vi "simulation.vi"(6 "stop":bool) -> ()   [LabVIEW 2010]
uses:
  red_tweezers_globals_INTERNAL.vi
  red_tweezers_globals.vi
  red_tweezers_globals_INTERNAL_VOLATILE.vi
  simulation_globals.vi
  <vilib>/Analysis/NI_AALBase.lvlib
panel:
  out "Image Out":T1(plugin-control)
  in  "timestep/s":dbl=0.009999999999999997 format="%.2p"
  in  "sedimentation velocity (m/s)":dbl=5e-07
  in  "trap autocorrelation time (s)":dbl=0.01
  in  "capture radius (m)":dbl=3e-06
  in  "diffusion (m/sqrt(s))":dbl=4e-07 format="%.2p"
  in  "Number of Particles":i32=10
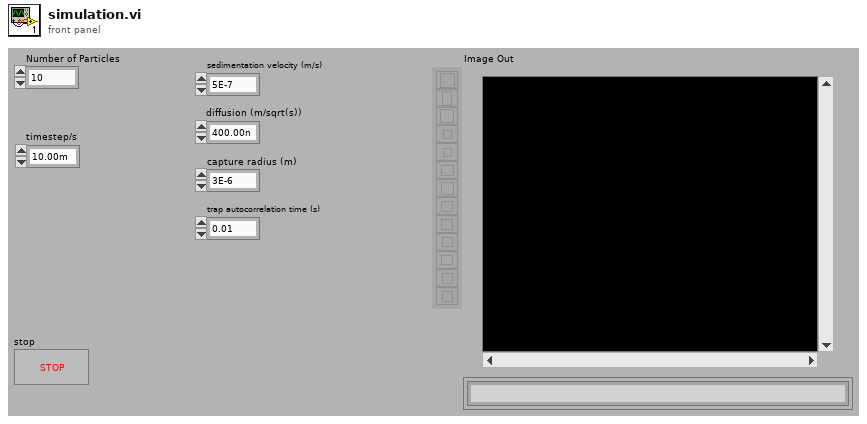
[diagram p1: front panel]
types:
  T1 = typedef "IMAQ Image.ctl" = refnum<image>
  T2 = enum32{"Bad", "Idle", "Run top level", "Running"}
  T3 = typedef "spot.ctl" = cluster{"Position":cluster{"x":dbl, "y":dbl, "z":dbl}, "Intensity":dbl, "Vortex Charge":i8, "Phase":dbl, "NA Position":cluster{"x":dbl, "y":dbl, "r":dbl}, "Line Trapping":T4, "Amplitude Correction":dbl}
  T4 = typedef "line_trapping.ctl" = cluster{"Vector":cluster{"x":dbl, "y":dbl, "z":dbl}, "Phase Gradient":dbl}
  T5 = cluster{"number: 0 to 1":dbl, "number: 0 to 1":dbl, "number: 0 to 1":dbl}
  T6 = cluster{"Gaussian noise pattern[0]":dbl, "Gaussian noise pattern[1]":dbl, "Gaussian noise pattern[2]":dbl}
  T7 = cluster{"capture radius":dbl, "capture radius":dbl, dbl}
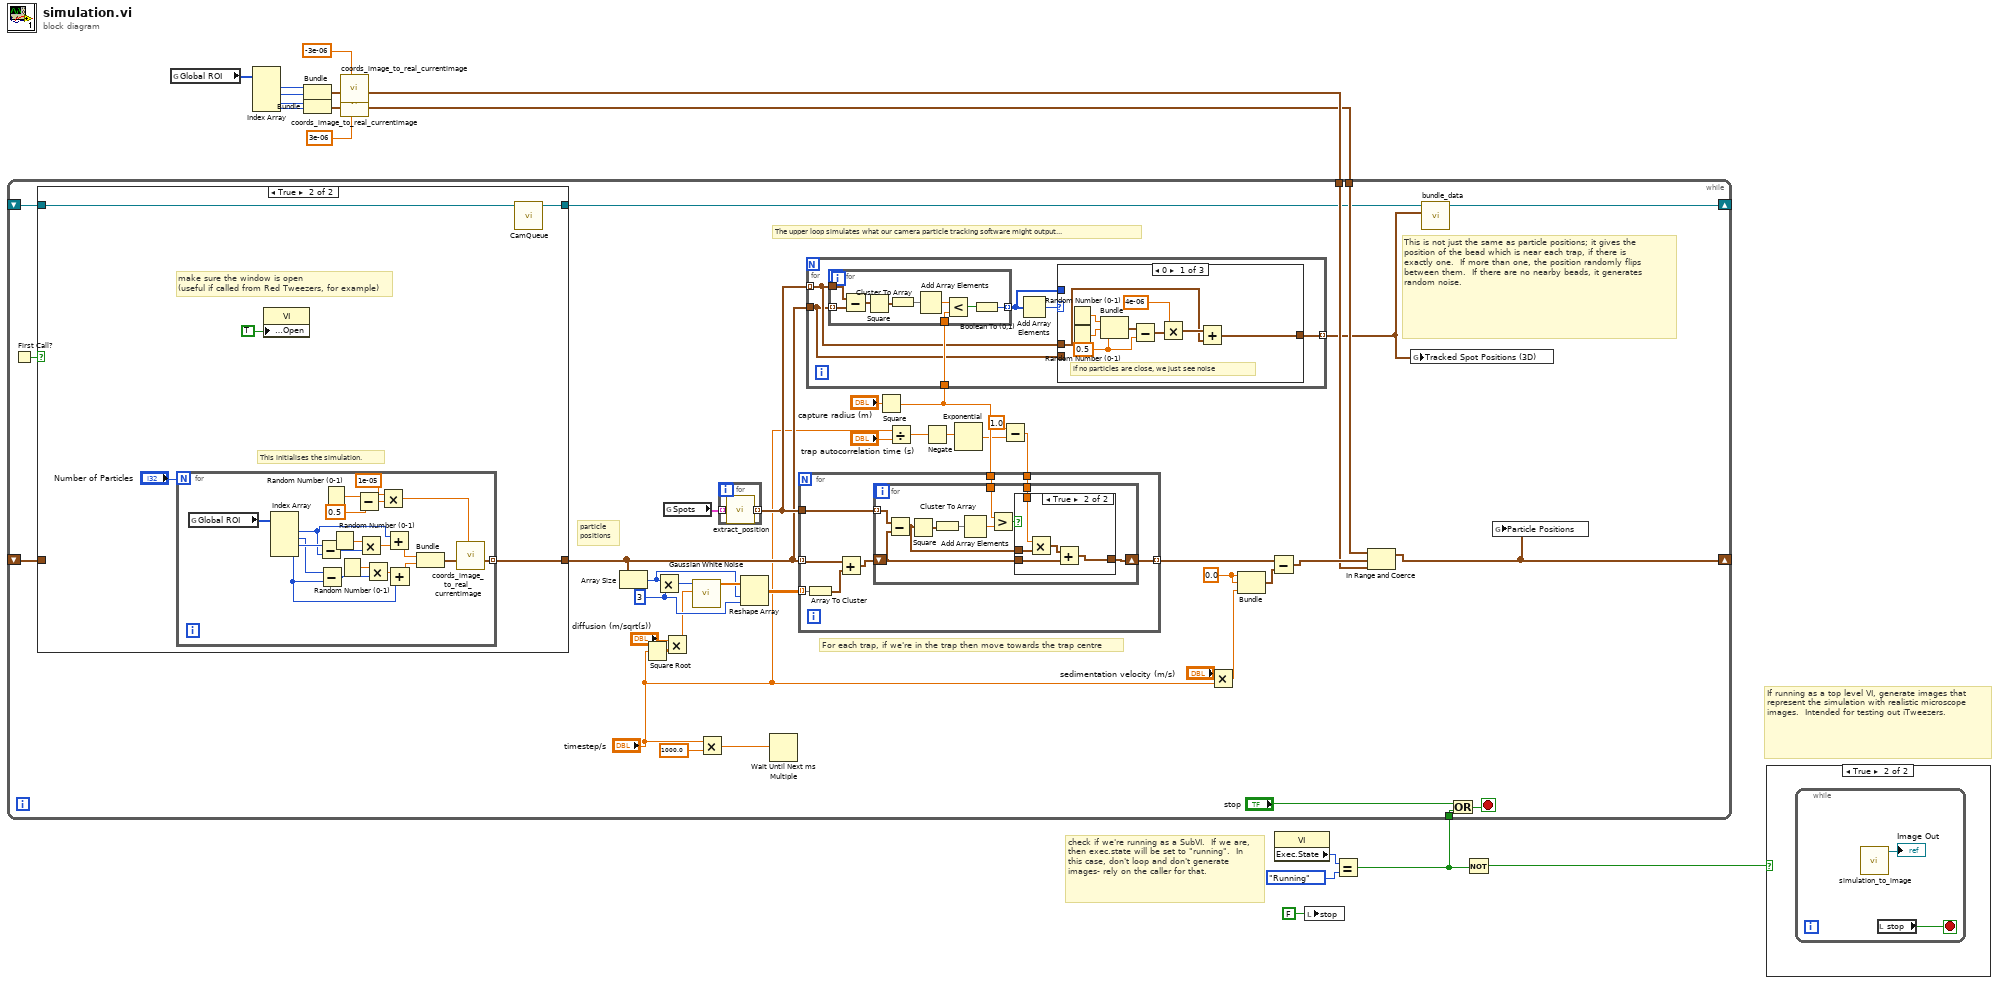
[diagram p0: block diagram]
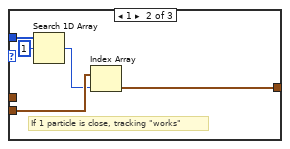
[diagram p4: hidden frame]
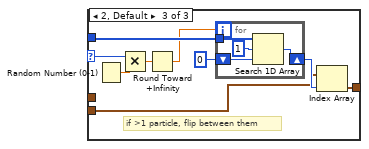
[diagram p5: hidden frame]
diagram:
  # "If running as a top level VI, generate images that represent the simulation with realistic microscope images.  Intended for testing out iTweezers."
  # "check if we're running as a SubVI.  If we are, then exec.state will be set to \"running\".  In this case, don't loop and don't generate images- rely on the caller for that."
  n1 = global read "red_tweezers_globals_INTERNAL.vi" "Global ROI"() -> (w16:i32[])
  n2 = Index Array(array=w16) -> (element #1=w15:i32, element #2=w14:i32, element #3=w9:i32, element #4=w8:i32)  [unwired: 4 in]
  n3 = Bundle("Numeric"=w15, "Numeric"=w14) -> (w13:cluster{"Numeric":i32, "Numeric":i32})  [unwired: 1 in]
  n4 = Bundle("Numeric"=w9, "Numeric"=w8) -> (w10:cluster{"Numeric":i32, "Numeric":i32})  [unwired: 1 in]
  n5 = call "coords_image_to_real_currentimage.vi"("Position (pixels on image)"=w13, "z (real coords)"=-3e-06) -> ("Position (real coords)"=w7:cluster{dbl, dbl, "Z":dbl})  [unwired: 8 in]
  n6 = call "coords_image_to_real_currentimage.vi"("Position (pixels on image)"=w10, "z (real coords)"=3e-06) -> ("Position (real coords)"=w6:cluster{dbl, dbl, "Z":dbl})  [unwired: 8 in]
  n7 = property class="VI"() -> ("Exec.State"=w5:T2)  [unwired: 2 in, 2 out]
  n8 = local write "stop"(FALSE ("stop")) -> ()
  n9 = Equal?(x=w5, y=T2."Running" ("Execution:State")) -> (x = y?=w2:bool)
  n10 = while {
    shift-right: [w44] -> _
    shift-left: _ -> [w29]
    tunnel: w7 -> [w43]
    tunnel: w6 -> [w42]
    shift-right: [w33] -> _
    shift-left: _ -> [w28]
    tunnel: w2 -> [w24]
    stop <- w26 stop-if-true
    w48 = 0.0 ("capture radius")
    w52 = 3 ("y")
    # "particle\npositions"
    # "This is not just the same as particle positions; it gives the position of the bead which is near each trap, if there is exactly one.  If more than one, the position randomly flips between them.  If there are no nearby beads, it generates random noise."
    # "The upper loop simulates what our camera particle tracking software might output..."
    # "For each trap, if we're in the trap then move towards the trap centre"
    n11 = First Call?() -> (First Call?: T/F=w27:bool)
    n12 = case shown="True" w27 {
      tunnel: [w57 w61] -> w30
      tunnel: [w56 w59] -> _
      tunnel: w29 -> [w57 _]
      tunnel: w28 -> [w56 _]
      frame False {
      }
      frame True {
        # "make sure the window is open\n(useful if called from Red Tweezers, for example)"
        # "This initialises the simulation."
        n13 = for {
          N: "Number of Particles" -> [_]
          tunnel: [w62] -> w61 mode=indexing
          n14 = global read "red_tweezers_globals_INTERNAL.vi" "Global ROI"() -> (w81:i32[])
          n15 = Index Array(array=w81) -> (element #1=w75:i32, element #2=w79:i32, element #3=w80:i32, element #4=w71:i32)  [unwired: 4 in]
          n16 = Subtract(x=w80, y=w75) -> (x-y=w78:i32)
          n17 = Subtract(x=w79, y=w71) -> (x-y=w73:i32)
          n18 = Random Number (0-1)() -> (number: 0 to 1=w67:dbl)
          n19 = Random Number (0-1)() -> (number: 0 to 1=w76:dbl)
          n20 = Random Number (0-1)() -> (number: 0 to 1=w74:dbl)
          n21 = Subtract(x=w67, y=0.5) -> (x-y=w65:dbl)
          n22 = Multiply(x=w76, y=w78) -> (x*y=w77:dbl)
          n23 = Multiply(x=w74, y=w73) -> (x*y=w72:dbl)
          n24 = Multiply(x=1e-05, y=w65) -> (x*y=w63:dbl)
          n25 = Add(x=w75, y=w77) -> (x+y=w69:dbl)
          n26 = Add(x=w72, y=w71) -> (x+y=w70:dbl)
          n27 = Bundle(w69, w70) -> (w68:cluster{dbl, dbl})  [unwired: 1 in]
          n28 = call "coords_image_to_real_currentimage.vi"("Position (pixels on image)"=w68, "z (real coords)"=w63) -> ("Position (real coords)"=w62:cluster{dbl, dbl, "Z":dbl})  [unwired: 8 in]
        }
        n29 = property class="VI"("Front Panel.Open"=TRUE ("Front Panel Window:Open")) -> ()  [unwired: 2 in, 2 out]
        n30 = call "CamQueue.vi"() -> ("queue out"=w59:refnum<queue>)  [unwired: 3 in]
      }
    }
    n31 = Array Size(array=w30) -> (size(s)=w53:i32)
    n32 = Square Root(x="timestep/s") -> (sqrt(x)=w39:dbl)
    n33 = Multiply(x=w53, y=w52) -> (x*y=w55:i32)
    n34 = Multiply(x="diffusion (m/sqrt(s))", y=w39) -> (x*y=w41:dbl)
    n35 = global read "red_tweezers_globals.vi" "Spots"() -> (w50:T3[])
    n36 = call <vilib>:"Gaussian White Noise.vi"("standard deviation"=w41, "samples"=w55) -> ("Gaussian noise pattern"=w54:dbl[])  [unwired: 8 in, 1 out]
    n37 = Multiply(x="timestep/s", y=1000.0) -> (x*y=w37:dbl)
    n38 = for {
      tunnel: w50 -> [w125] mode=indexing
      tunnel: [w124] -> w35 mode=indexing
      n39 = call "extract_position.vi"("Spot"=w125) -> ("Position"=w124:cluster{"x":dbl, "y":dbl, "z":dbl})
    }
    n40 = Reshape Array(w54, w53, w52) -> (w51:dbl[][])
    n41 = Wait Until Next ms Multiple(millisecond multiple=w37) -> ()  [unwired: 1 out]
    n42 = Square(x="capture radius (m)") -> (x^2=w31:dbl)
    n43 = for {
      tunnel: w35 -> [w85] mode=indexing
      tunnel: w30 -> [w84]
      tunnel: w31 -> [w87]
      tunnel: [w82] -> w32 mode=indexing
      n44 = for {
        tunnel: w85 -> [w123]
        tunnel: w84 -> [w118] mode=indexing
        tunnel: w87 -> [w117]
        tunnel: [w115] -> w83 mode=indexing
        n45 = Subtract(x=w123, y=w118) -> (x-y=w119:cluster{dbl, dbl, dbl})
        n46 = Square(x=w119) -> (x^2=w122:cluster{dbl, dbl, dbl})
        n47 = Cluster To Array(cluster=w122) -> (array=w121:dbl[])
        n48 = Add Array Elements(numeric array=w121) -> (sum=w120:dbl)
        n49 = Less?(x=w120, y=w117) -> (x < y?=w116:bool)
        n50 = Boolean To (0,1)(Boolean=w116) -> (0, 1=w115:i16)
      }
      n51 = Add Array Elements(numeric array=w83) -> (sum=w86:i16)
      n52 = case shown="0" w86 {
        selector: w86 -> [_ _ w109]
        tunnel: w85 -> [w88 _ _]
        tunnel: w84 -> [_ w101 w102]
        tunnel: [w89 w97 w103] -> w82
        tunnel: w83 -> [_ w100 w107]
        frame 0 {
          w94 = 0.5 ("number: 0 to 1")
          # "if no particles are close, we just see noise"
          n53 = Random Number (0-1)() -> (number: 0 to 1=w96:dbl)
          n54 = Random Number (0-1)() -> (number: 0 to 1=w95:dbl)
          n55 = Bundle("number: 0 to 1"=w96, "number: 0 to 1"=w95, "number: 0 to 1"=w94) -> (w91:T5)  [unwired: 1 in]
          n56 = Subtract(x=w91, y=w94) -> (x-y=w93:T5)
          n57 = Multiply(x=4e-06, y=w93) -> (x*y=w90:T5)
          n58 = Add(x=w90, y=w88) -> (x+y=w89:cluster{dbl, dbl, dbl})
        }
        frame 1 {
          # "If 1 particle is close, tracking \"works\""
          n59 = Search 1D Array(1D array=w100, element=i16 1) -> (index of element=w98:i32)  [unwired: 1 in]
          n60 = Index Array(array=w101, index=w98) -> (element=w97:cluster{dbl, dbl, "Z":dbl})
        }
        frame 2, Default {
          # "if >1 particle, flip between them"
          n61 = Random Number (0-1)() -> (number: 0 to 1=w110:dbl)
          n62 = Multiply(x=w109, y=w110) -> (x*y=w108:dbl)
          n63 = Round Toward +Infinity(x=w108) -> (ceil(x): smallest int >= x=w106:dbl)
          n64 = for {
            N: w106 -> [_]
            tunnel: w107 -> [w114]
            shift-right: [w112] -> w104
            shift-left: 0 ("index of element") -> [w111]
            n65 = Search 1D Array(1D array=w114, element=i16 1, start index (0)=w111) -> (index of element=w112:i32)
          }
          n66 = Index Array(array=w102, index=w104) -> (element=w103:cluster{dbl, dbl, "Z":dbl})
        }
      }
    }
    n67 = Divide(x="timestep/s", y="trap autocorrelation time (s)") -> (x/y=w22:dbl)
    n68 = Negate(x=w22) -> (-x=w17:dbl)
    n69 = Exponential(1:w17) -> (0:w23:dbl)
    n70 = Subtract(x=1.0 ("y"), y=w23) -> (x-y=w19:dbl)
    n71 = for {
      tunnel: w30 -> [w132] mode=indexing
      tunnel: w51 -> [w133] mode=indexing
      tunnel: w35 -> [w130]
      tunnel: w31 -> [w128]
      tunnel: w19 -> [w127]
      tunnel: [w126] -> w49 mode=indexing
      n72 = Array To Cluster(array=w133) -> (cluster=w131:T6)
      n73 = Add(x=w132, y=w131) -> (x+y=w129:cluster{dbl, dbl, dbl})
      n74 = for {
        tunnel: w130 -> [w143] mode=indexing
        tunnel: w128 -> [w139]
        shift-right: [w134] -> w126
        shift-left: w129 -> [w135]
        tunnel: w127 -> [w136]
        n75 = Subtract(x=w143, y=w135) -> (x-y=w137:cluster{dbl, dbl, dbl})
        n76 = Square(x=w137) -> (x^2=w142:cluster{dbl, dbl, dbl})
        n77 = Cluster To Array(cluster=w142) -> (array=w141:dbl[])
        n78 = Add Array Elements(numeric array=w141) -> (sum=w140:dbl)
        n79 = Greater?(x=w139, y=w140) -> (0:w138:bool)
        n80 = case shown="True" w138 {
          tunnel: w137 -> [_ w149]
          tunnel: w136 -> [_ w148]
          tunnel: w135 -> [w144 w147]
          tunnel: [w144 w145] -> w134
          frame False {
          }
          frame True {
            n81 = Multiply(x=w148, y=w149) -> (x*y=w146:cluster{dbl, dbl, dbl})
            n82 = Add(x=w146, y=w147) -> (x+y=w145:cluster{dbl, dbl, dbl})
          }
        }
      }
    }
    n83 = Multiply(x="sedimentation velocity (m/s)", y="timestep/s") -> (x*y=w38:dbl)
    n84 = Bundle("capture radius"=w48, "capture radius"=w48, w38) -> (w46:T7)  [unwired: 1 in]
    n85 = Subtract(x=w49, y=w46) -> (x-y=w45:cluster{dbl, dbl, dbl}[])
    n86 = In Range and Coerce(upper limit=w42, x=w45, lower limit=w43) -> (coerced(x)=w44:cluster{dbl, dbl, "Z":dbl}[])  [unwired: 1 out]
    n87 = global write "red_tweezers_globals_INTERNAL_VOLATILE.vi" "Tracked Spot Positions (3D)"(w32) -> ()
    n88 = call "bundle_data.vi"("Array"=w32, "queue"=w28) -> ("queue out"=w33:refnum<queue>)  [unwired: 4 in, 1 out]
    n89 = Or(x="stop", y=w24) -> (x .or. y?=w26:bool)
    n90 = global write "simulation_globals.vi" "Particle Positions"(w44) -> ()
  }
  n91 = Not(x=w2) -> (.not. x?=w1:bool)
  n92 = case shown="True" w1 {
    frame False {
    }
    frame True {
      n93 = while {
        stop <- w151 stop-if-true
        n94 = call "simulation_to_image.vi"() -> ("Image Out"=→"Image Out":T1)  [unwired: 11 in]
        n95 = local read "stop"() -> (w151:bool)
      }
    }
  }
